vi "测量数据区.vi"(11 "数组":u16[](array[numeric]) format="%04xH") -> (3 "测量数据区":T1 {"单位" items=["ug/L", "mg/L", "ppm", "mg/m3", "cm", "ppb", "ug/m3", "%", "nmol/mol", "umol/mol", "MPN/L", "MPN/100ml", "ng/m3", "NTU", "无量纲", "ms/cm", "us/cm", "℃", "mV", "万个/L"]})   [LabVIEW 2022 SP3, in "挥发酚.lvlib"]
panel:
  # "共占用105 WORD"
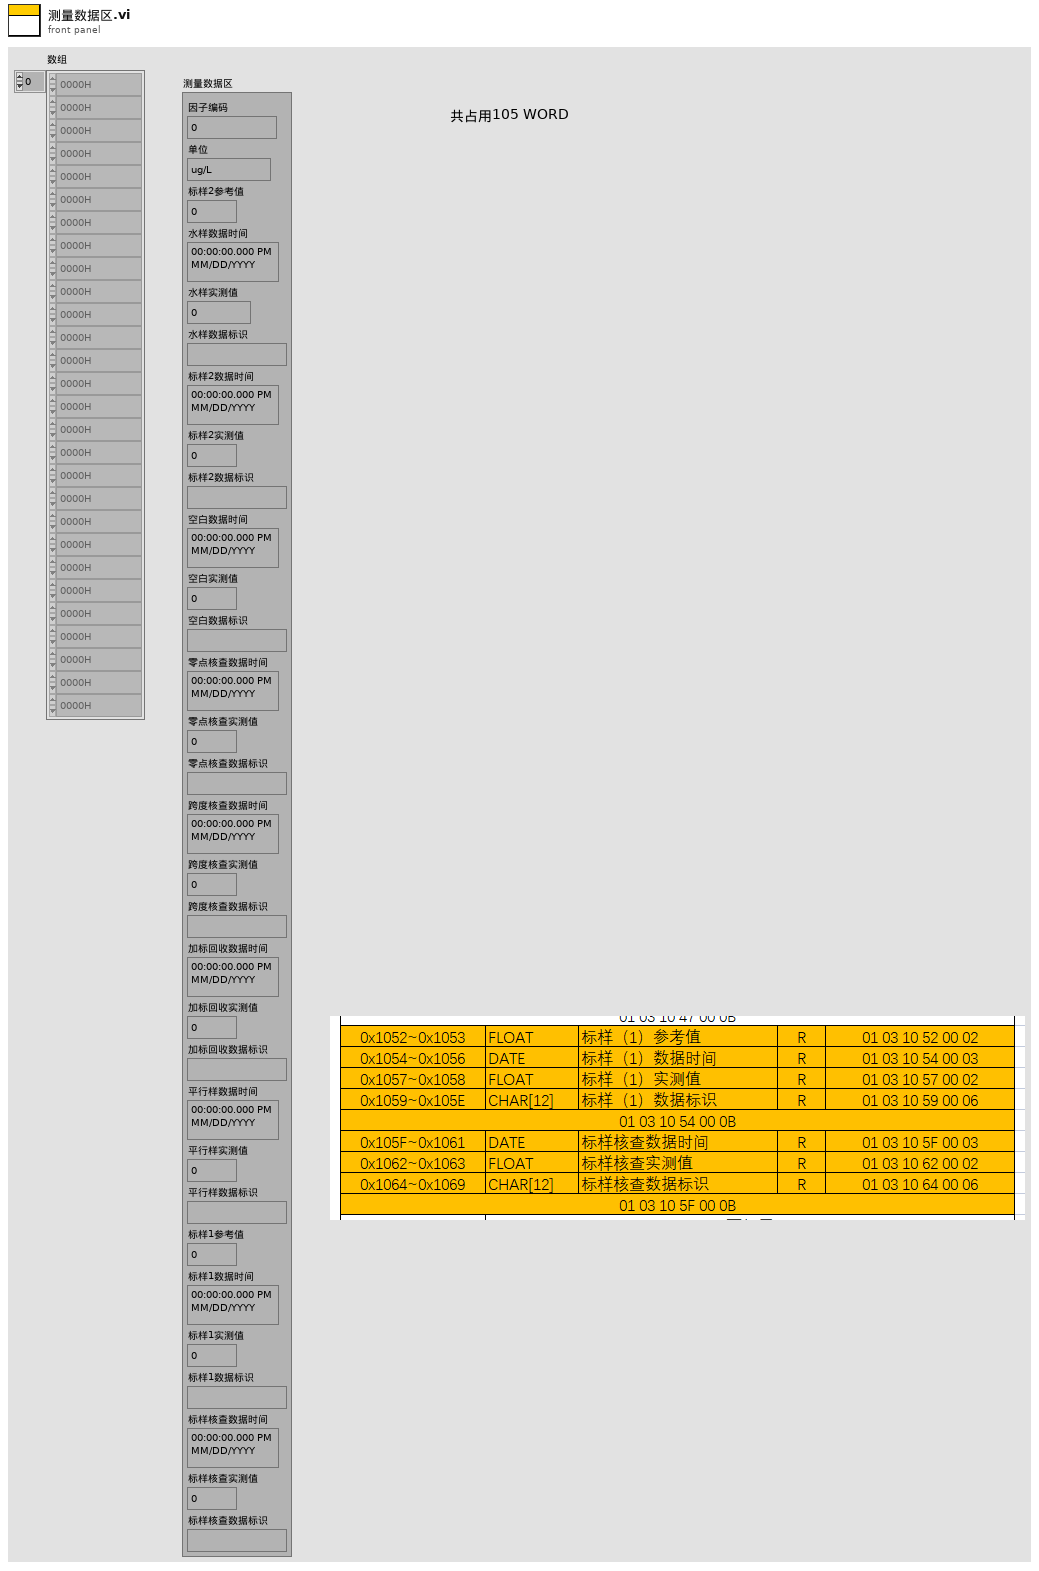
[diagram p1: front panel]
types:
  T1 = cluster{"因子编码":u32, "单位":u16, "标样2参考值":sgl, "水样数据时间":timestamp, "水样实测值":sgl, "水样数据标识":string, "标样2数据时间":timestamp, "标样2实测值":sgl, "标样2数据标识":string, "空白数据时间":timestamp, "空白实测值":sgl, "空白数据标识":string, "零点核查数据时间":timestamp, "零点核查实测值":sgl, "零点核查数据标识":string, "跨度核查数据时间":timestamp, "跨度核查实测值":sgl, "跨度核查数据标识":string, "加标回收数据时间":timestamp, "加标回收实测值":sgl, "加标回收数据标识":string, "平行样数据时间":timestamp, "平行样实测值":sgl, "平行样数据标识":string, "标样1参考值":sgl, "标样1数据时间":timestamp, "标样1实测值":sgl, "标样1数据标识":string, "标样核查数据时间":timestamp, "标样核查实测值":sgl, "标样核查数据标识":string}
  T2 = cluster{"系统时间":timestamp, "工作状态":u16, "测量模式":enum16{"待机", "连续模式", "周期模式", "定点模式", "受控模式", "手动模式"}, "告警代码":u16, "故障代码":u16, "日志代码":u16, "软件版本":u16, "测量间隔":u16, "消解实时温度":dbl, "校准间隔（天）":u16, "校准间隔（时）":u16, "周期测量时间（23_16）":u16, "周期测量时间（15_0）":u16, "清洗周期（次数）":u16, "运行模式":u16, "自动校准状态":u16, "自动清洗状态":u16}
  T3 = cluster{"水样数据时间":timestamp, "空白数据时间":timestamp, "零点核查数据时间":timestamp, "跨度核查数据时间":timestamp, "加标回收数据时间":timestamp, "平行样数据时间":timestamp, "标样核查数据时间":timestamp, "标样1数据时间":timestamp, "标样2数据时间":timestamp}
  T4 = cluster{"WORD":u16, "WORD":u16, "FLOAT":sgl, "time stamp":timestamp, "数值":sgl, "string":string, "time stamp":timestamp, "数值":sgl, "string":string, "time stamp":timestamp, "数值":sgl, "string":string, "time stamp":timestamp, "数值":sgl, "string":string, "time stamp":timestamp, "数值":sgl, "string":string, "time stamp":timestamp, "数值":sgl, "string":string, "time stamp":timestamp, "数值":sgl, "string":string, "FLOAT":sgl, "time stamp":timestamp, "数值":sgl, "string":string, "time stamp":timestamp, "数值":sgl, "string":string}
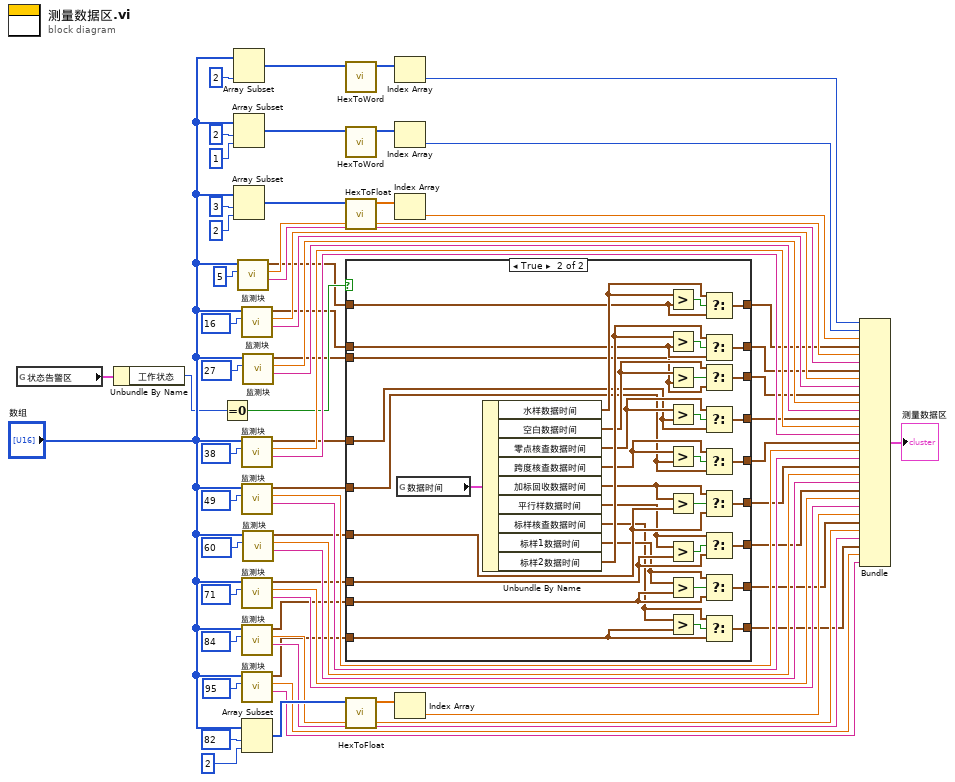
[diagram p0: block diagram]
diagram:
  n1 = global read "VAR挥发酚全局变量.vi" "状态告警区"() -> (w21:T2)
  n2 = Unbundle By Name(w21) -> ("工作状态"=w20:u16)
  n3 = Equal To 0?(x=w20) -> (x = 0?=w19:bool)
  n4 = Array Subset(array="数组", length=2 ("长度")) -> (w35:u16[])  [unwired: 1 in]
  n5 = Array Subset(array="数组", index=2 ("索引"), length=1 ("长度")) -> (w66:u16[])
  n6 = Array Subset(array="数组", index=3 ("索引"), length=2 ("长度")) -> (w61:u16[])
  n7 = call "监测块.vi"("索引"=5, "数组"="数组") -> ("string"=w57:string, "数值"=w58:sgl, "time stamp"=w18:timestamp)  [unwired: 7 in]
  n8 = call "监测块.vi"("索引"=16, "数组"="数组") -> ("string"=w53:string, "数值"=w54:sgl, "time stamp"=w16:timestamp)  [unwired: 7 in]
  n9 = call "监测块.vi"("索引"=38, "数组"="数组") -> ("string"=w47:string, "数值"=w48:sgl, "time stamp"=w13:timestamp)  [unwired: 7 in]
  n10 = call "监测块.vi"("索引"=49, "数组"="数组") -> ("string"=w44:string, "数值"=w45:sgl, "time stamp"=w10:timestamp)  [unwired: 7 in]
  n11 = call "监测块.vi"("索引"=71, "数组"="数组") -> ("string"=w38:string, "数值"=w39:sgl, "time stamp"=w6:timestamp)  [unwired: 7 in]
  n12 = call "监测块.vi"("索引"=84, "数组"="数组") -> ("string"=w24:string, "数值"=w25:sgl, "time stamp"=w4:timestamp)  [unwired: 7 in]
  n13 = call "监测块.vi"("索引"=95, "数组"="数组") -> ("string"=w22:string, "数值"=w23:sgl, "time stamp"=w2:timestamp)  [unwired: 7 in]
  n14 = Array Subset(array="数组", index=82 ("索引"), length=2 ("长度")) -> (w30:u16[])
  n15 = call "监测块.vi"("索引"=27, "数组"="数组") -> ("string"=w50:string, "数值"=w51:sgl, "time stamp"=w14:timestamp)  [unwired: 7 in]
  n16 = call "监测块.vi"("索引"=60, "数组"="数组") -> ("string"=w41:string, "数值"=w42:sgl, "time stamp"=w8:timestamp)  [unwired: 7 in]
  n17 = call "HexToWord.vi"("数组"=w35) -> ("WORD"=w34:u16[])  [unwired: 10 in]
  n18 = call "HexToWord.vi"("数组"=w66) -> ("WORD"=w65:u16[])  [unwired: 10 in]
  n19 = call "HexToFloat.vi"("数组"=w61) -> ("FLOAT"=w60:sgl[])  [unwired: 10 in]
  n20 = case shown="True" w19 {
    tunnel: w18 -> [w78 w112]
    tunnel: [w78 w111] -> w17
    tunnel: w16 -> [w77 w108]
    tunnel: [w77 w107] -> w15
    tunnel: w14 -> [w76 w104]
    tunnel: [w76 w103] -> w11
    tunnel: w13 -> [w75 w100]
    tunnel: [w75 w99] -> w12
    tunnel: w10 -> [w74 w96]
    tunnel: [w74 w95] -> w9
    tunnel: w8 -> [w73 w92]
    tunnel: [w73 w91] -> w7
    tunnel: w6 -> [w72 w88]
    tunnel: [w72 w87] -> w5
    tunnel: w4 -> [w71 w84]
    tunnel: [w71 w83] -> w3
    tunnel: w2 -> [w70 w81]
    tunnel: [w70 w79] -> w1
    frame False {
    }
    frame True {
      n21 = global read "挥发酚断电保存全局变量.vi" "数据时间"() -> (w115:T3)
      n22 = Unbundle By Name(w115) -> ("水样数据时间"=w113:timestamp, "空白数据时间"=w105:timestamp, "零点核查数据时间"=w101:timestamp, "跨度核查数据时间"=w97:timestamp, "加标回收数据时间"=w93:timestamp, "平行样数据时间"=w89:timestamp, "标样核查数据时间"=w80:timestamp, "标样1数据时间"=w85:timestamp, "标样2数据时间"=w109:timestamp)
      n23 = Greater?(x=w113, y=w112) -> (0:w114:bool)
      n24 = Greater?(x=w109, y=w108) -> (0:w110:bool)
      n25 = Greater?(x=w105, y=w104) -> (0:w106:bool)
      n26 = Greater?(x=w101, y=w100) -> (0:w102:bool)
      n27 = Greater?(x=w97, y=w96) -> (0:w98:bool)
      n28 = Greater?(x=w93, y=w92) -> (0:w94:bool)
      n29 = Greater?(x=w89, y=w88) -> (0:w90:bool)
      n30 = Greater?(x=w85, y=w84) -> (0:w86:bool)
      n31 = Greater?(x=w80, y=w81) -> (0:w82:bool)
      n32 = Select(t=w113, s=w114, f=w112) -> (s? t:f=w111:timestamp)
      n33 = Select(t=w109, s=w110, f=w108) -> (s? t:f=w107:timestamp)
      n34 = Select(t=w105, s=w106, f=w104) -> (s? t:f=w103:timestamp)
      n35 = Select(t=w101, s=w102, f=w100) -> (s? t:f=w99:timestamp)
      n36 = Select(t=w97, s=w98, f=w96) -> (s? t:f=w95:timestamp)
      n37 = Select(t=w93, s=w94, f=w92) -> (s? t:f=w91:timestamp)
      n38 = Select(t=w89, s=w90, f=w88) -> (s? t:f=w87:timestamp)
      n39 = Select(t=w85, s=w86, f=w84) -> (s? t:f=w83:timestamp)
      n40 = Select(t=w80, s=w82, f=w81) -> (s? t:f=w79:timestamp)
    }
  }
  n41 = call "HexToFloat.vi"("数组"=w30) -> ("FLOAT"=w31:sgl[])  [unwired: 10 in]
  n42 = Index Array(array=w34) -> (element=w37:u16)  [unwired: 1 in]
  n43 = Index Array(array=w65) -> (element=w64:u16)  [unwired: 1 in]
  n44 = Index Array(array=w60) -> (element=w59:sgl)  [unwired: 1 in]
  n45 = Index Array(array=w31) -> (element=w27:sgl)  [unwired: 1 in]
  n46 = Bundle("WORD"=w37, "WORD"=w64, "FLOAT"=w59, "time stamp"=w17, "数值"=w58, "string"=w57, "time stamp"=w15, "数值"=w54, "string"=w53, "time stamp"=w11, "数值"=w51, "string"=w50, "time stamp"=w12, "数值"=w48, "string"=w47, "time stamp"=w9, "数值"=w45, "string"=w44, "time stamp"=w7, "数值"=w42, "string"=w41, "time stamp"=w5, "数值"=w39, "string"=w38, "FLOAT"=w27, "time stamp"=w3, "数值"=w25, "string"=w24, "time stamp"=w1, "数值"=w23, "string"=w22) -> (→"测量数据区":T4)  [unwired: 1 in]
